vi "Renew UI Attributes From Configuration.vi"(8 "error in (no error)":errorcluster, 10 "section":string="ScriptsDialog", 11 "ScriptDialog in":refnum<class "ScriptDialog.lvclass">) -> (0 "error out":errorcluster, 3 "ScriptDialog out":refnum<class "ScriptDialog.lvclass">)   [LabVIEW 2015, in "ScriptDialog.lvclass"]
uses:
  ScriptDialog.lvclass
  ScriptDialog.lvclass/ScriptDialog.ctl
  System/UIConfiguration/UIConfiguration.lvclass
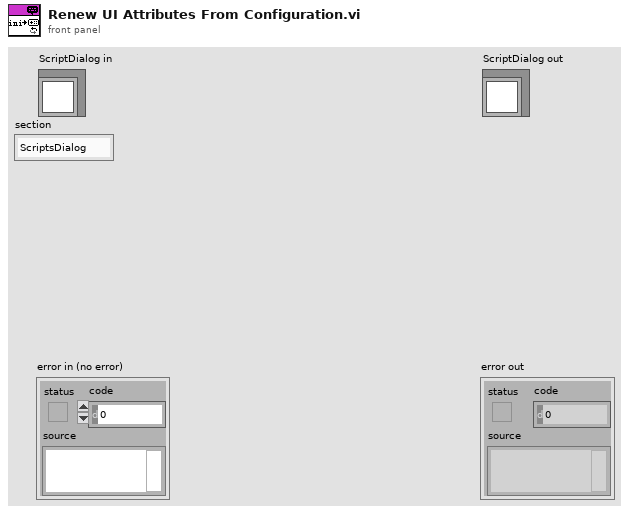
[diagram p1: front panel]
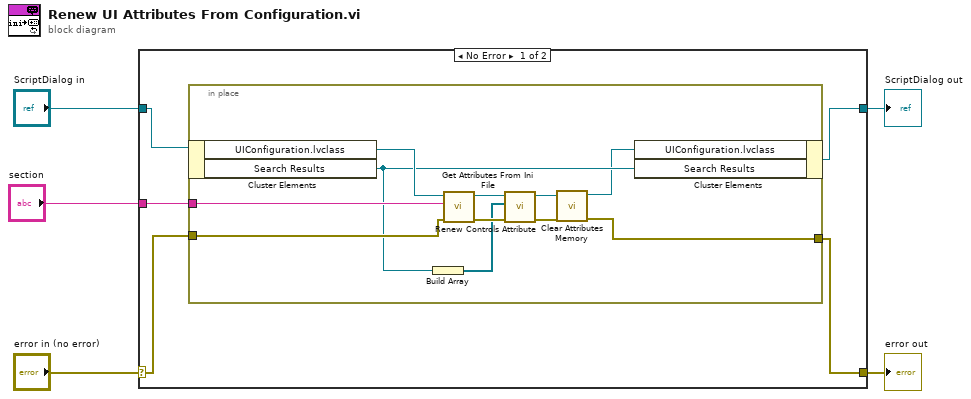
[diagram p0: block diagram]
diagram:
  n1 = case shown="No Error" "error in (no error)" {
    selector: "error in (no error)" -> [w9 w23]
    tunnel: [w6 w23] -> w4
    tunnel: [w7 w22] -> w2
    tunnel: "ScriptDialog in" -> [w8 w22]
    tunnel: "section" -> [w10 _]
    frame No Error {
      n2 = in-place {
        in-place-border: w10 -> [w21]
        in-place-border: w9 -> [w20]
        in-place-border: [w11] -> w6
        n3 = in-place-cluster #1(w8) -> ("UIConfiguration.lvclass"=w17:refnum<class "UIConfiguration.lvclass">, "Search Results"=w16:refnum<vi>)
        n4 = Build Array(w16) -> (w15:refnum<vi>[])
        n5 = call "Get Attributes From Ini File.vi"("error in (no error)"=w20, "section"=w21, "UIConfiguration in"=w17) -> ("error out"=w18:errorcluster, "UIConfiguration out"=w19:refnum<class "UIConfiguration.lvclass">)  [unwired: 7 in]
        n6 = call-dynamic "Renew Controls Attribute.vi"("error in (no error)"=w18, "Control Refs"=w15, "UIConfiguration in"=w19) -> ("error out"=w13:errorcluster, "UIConfiguration out"=w14:refnum<class "UIConfiguration.lvclass">)  [unwired: 7 in]
        n7 = call "Clear Attributes Memory.vi"("error in (no error)"=w13, "UIConfiguration in"=w14) -> ("error out"=w11:errorcluster, "UIConfiguration out"=w12:refnum<class "UIConfiguration.lvclass">)  [unwired: 8 in]
        n8 = in-place-cluster #1("UIConfiguration.lvclass"=w12, "Search Results"=w16) -> (w7:refnum<class "ScriptDialog.lvclass">)
      }
    }
    frame Error {
    }
  }
  "error out" <- w4
  "ScriptDialog out" <- w2
